vi "MB ICPCON Param Read timeout.vi"(7 "Param Reference":T2, 8 "error in (no error)":errorcluster, 11 "N":i32) -> (0 "error out":errorcluster, 1 "timeout":T1={"conn_timeout"=1000, "reconn_timeout"=0, "N attempt max"=3, "t_reset_TTL"=120000, "write_timeout"=50, "read_timeout"=500, "period"=100})   [LabVIEW 2019, in "ICPCON_Param.lvlib"]
uses:
  ICPCON_Param.lvlib
  ICPCON Param.ctl
  Eth timeouts.ctl
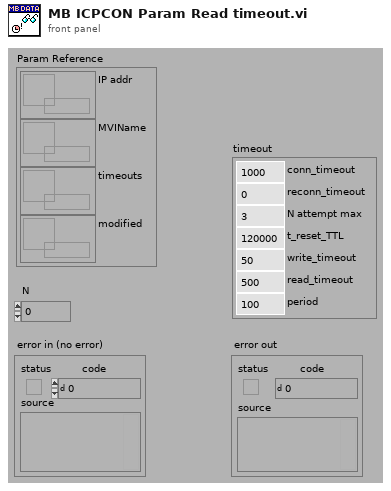
[diagram p1: front panel]
types:
  T1 = typedef "ICPCON_Param.lvlib/Eth timeouts.ctl" = cluster{"conn_timeout":i32, "reconn_timeout":i32, "N attempt max":i32, "t_reset_TTL":i32, "write_timeout":i32, "read_timeout":i32, "period":i32}
  T2 = typedef "ICPCON_Param.lvlib/ICPCON Param.ctl" = cluster{"IP addr":refnum<data-value>, "MVIName":refnum<data-value>, "timeouts":refnum<data-value>, "modified":refnum<data-value>}
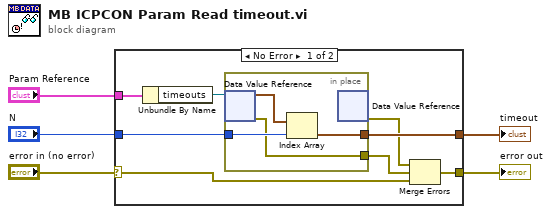
[diagram p0: block diagram]
diagram:
  n1 = case shown="No Error" "error in (no error)" {
    selector: "error in (no error)" -> [w6 w18]
    tunnel: [w10 w18] -> w5
    tunnel: [w13 _] -> w2
    tunnel: "N" -> [w12 _]
    tunnel: "Param Reference" -> [w11 _]
    frame No Error {
      n2 = Unbundle By Name(w11) -> ("timeouts"=w7:refnum<data-value>)
      n3 = in-place {
        in-place-border: w12 -> [w17]
        in-place-border: [w15] -> w13
        in-place-border: [w14] -> w8
        n4 = in-place-dvr #1(w7) -> (w16:T1[], w14:errorcluster)
        n5 = Index Array(array=w16, index=w17) -> (element=w15:T1)
        n6 = in-place-dvr #1() -> (w9:errorcluster)  [unwired: 1 in, 1 out]
      }
      n7 = Merge Errors(w9, w8, w6) -> (w10:errorcluster)
    }
    frame Error {
    }
  }
  "error out" <- w5
  "timeout" <- w2
